vi "Destroy.vi"(0 "reference in":refnum<class "PauseButton.lvclass">, 11 "Error In":errorcluster) -> (4 "reference out":refnum<class "PauseButton.lvclass">, 15 "Error Out":errorcluster)   [LabVIEW 2024, in "PauseButton.lvclass"]
uses:
  PauseButton.lvclass/PauseButton.ctl
  PauseButton.lvclass
  Button_class/Button.lvclass
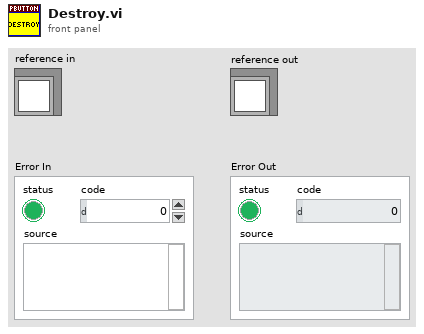
[diagram p1: front panel]
types:
  T1 = typedef "G4SubTemplate_Simple_5x6x5.lvclass/ObjectAttributes.ctl" = cluster{"Attribute1":dbl}
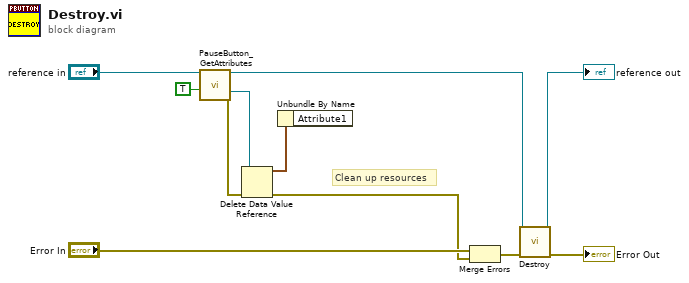
[diagram p0: block diagram]
diagram:
  # "Clean up resources"
  n1 = call "PauseButton_GetAttributes.vi"("reference in"="reference in", "OnlyGetDvrReference(False)"=TRUE) -> ("reference out"=w5:refnum<class "PauseButton.lvclass">, "DataRef"=w10:refnum<data-value>, "Error Out"=w11:errorcluster)  [unwired: 10 in, 1 out]
  n2 = Delete Data Value Reference(data value reference=w10, error in=w11) -> (data value=w1:T1, error out=w8:errorcluster)
  n3 = Unbundle By Name(w1) -> ()  [unwired: 1 out]
  n4 = Merge Errors("Error In", w8) -> (w6:errorcluster)
  n5 = call-parent "Destroy.vi"("reference in"=w5, "Error In"=w6) -> ("reference out"=→"reference out":refnum<class "PauseButton.lvclass">, "Error Out"=→"Error Out":errorcluster)  [unwired: 12 in]
